vi "DAQ_Stop_Tasks.vi"(8 "error in":errorcluster caption="entrée d'erreur", 11 "Cluster tasks":T1) -> (0 "error out":errorcluster, 3 "Cluster tasks OUT":T1)   [LabVIEW 2026]
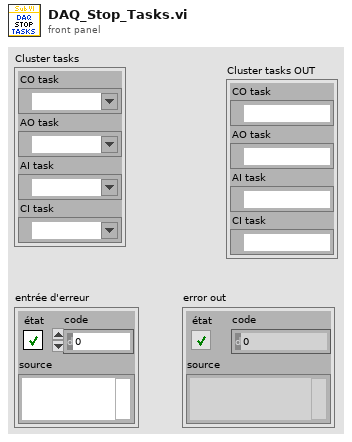
[diagram p1: front panel]
types:
  T1 = cluster{"CO task":refnum<k21>, "AO task":refnum<k21>, "AI task":refnum<k21>, "CI task":refnum<k21>}
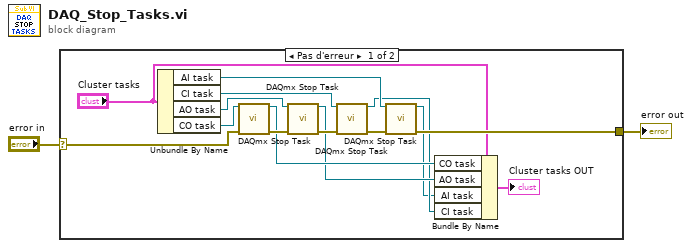
[diagram p0: block diagram]
diagram:
  n1 = case shown="Pas d'erreur" "error in" {
    selector: "error in" -> [w11 w18]
    tunnel: [w10 w18] -> w1
    frame No Error {
      n2 = Unbundle By Name("Cluster tasks") -> ("AI task"=w12:refnum<k21>, "CI task"=w13:refnum<k21>, "AO task"=w9:refnum<k21>, "CO task"=w14:refnum<k21>)
      n3 = call <vilib>:"DAQmx Stop Task.vi"("task/channels in"=w14, "error in"=w11) -> ("task out"=w7:refnum<k21>, "error out"=w15:errorcluster)  [unwired: 12 in]
      n4 = call <vilib>:"DAQmx Stop Task.vi"("task/channels in"=w9, "error in"=w15) -> ("task out"=w6:refnum<k21>, "error out"=w16:errorcluster)  [unwired: 12 in]
      n5 = call <vilib>:"DAQmx Stop Task.vi"("task/channels in"=w13, "error in"=w16) -> ("task out"=w5:refnum<k21>, "error out"=w17:errorcluster)  [unwired: 12 in]
      n6 = call <vilib>:"DAQmx Stop Task.vi"("task/channels in"=w12, "error in"=w17) -> ("task out"=w4:refnum<k21>, "error out"=w10:errorcluster)  [unwired: 12 in]
      n7 = Bundle By Name(cluster="Cluster tasks", "CO task"=w7, "AO task"=w6, "AI task"=w4, "CI task"=w5) -> (→"Cluster tasks OUT":T1)
    }
    frame Error {
    }
  }
  "error out" <- w1
